vi "UDT_admittanceLibrary_PID.vi"() -> (3 "Unit Test Framework Results":T1)   [LabVIEW 2017]
doc: "Use this template to create a user-defined test VI. Define your test requirements and wire the results to the <b>Result (Test)</b> control. Do not modify the <b>Unit Test Framework Results</b> indicator."
uses:
  <vilib>/utf/common/utf_test_result_troll.ctl
  <vilib>/utf/common/utf_test_result.ctl
  <vilib>/utf/common/utf_test_result_failure.ctl
  <vilib>/utf/common/utf_test_comparison_operators.ctl
  <vilib>/utf/common/utf_vi_tag.ctl
  <vilib>/Control Software Solutions Ltd/UTF Helper/SubVIs/UTF Boolean Equals.vi
  <vilib>/Control Software Solutions Ltd/UTF Helper/SubVIs/UTF Double Equals.vi
  <vilib>/Control Software Solutions Ltd/UTF Helper/Unit Test Helper.lvlib
  RT/Admittance Controller/admittanceControllerLibrary.lvlib
  <vilib>/utf/NI_UnitTestFramework.lvlib
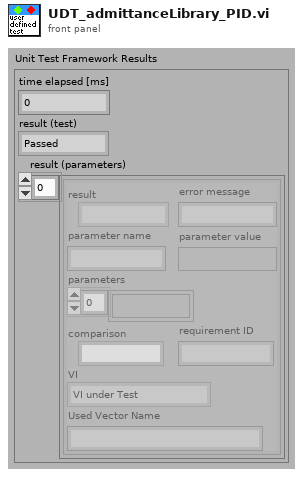
[diagram p1: front panel]
types:
  T1 = typedef "NI_UnitTestFramework.lvlib/utf_test_result_troll.ctl" = cluster{"time elapsed [ms]":u32, "result (test)":T2, "result (parameters)":T3[]}
  T2 = typedef "NI_UnitTestFramework.lvlib/utf_test_result.ctl" = enum16{"Passed", "Failed", "Error", "Skipped", "Not Processed"}
  T3 = typedef "NI_UnitTestFramework.lvlib/utf_test_result_failure.ctl" = cluster{"result":T2, "error message":string, "parameter name":string, "parameter value":variant, "parameters":variant[], "comparison":T4, "requirement ID":string, "VI":T5, "Used Vector Name":string}
  T4 = typedef "NI_UnitTestFramework.lvlib/utf_test_comparison_operators.ctl" = enum16{"=", "!=", ">", ">=", "<", "<=", "range", "symmetric tolerance", "asymmetric tolerance", "string contains", "string not contain", "array size", "string length", "array range", "by element", "array range (limit array)", "user-defined", "array contains", "array not contain", "vector length", "= (elm)", "!= (elm)", "= (case insensitive)", "!= (case insensitive)"}
  T5 = typedef "NI_UnitTestFramework.lvlib/utf_vi_tag.ctl" = enum16{"Setup VI", "VI under Test", "Teardown VI"}
  T6 = cluster{"proportional gain (Kc)":dbl, "integral time (Ti, min)":dbl, "derivative time (Td, min)":dbl}
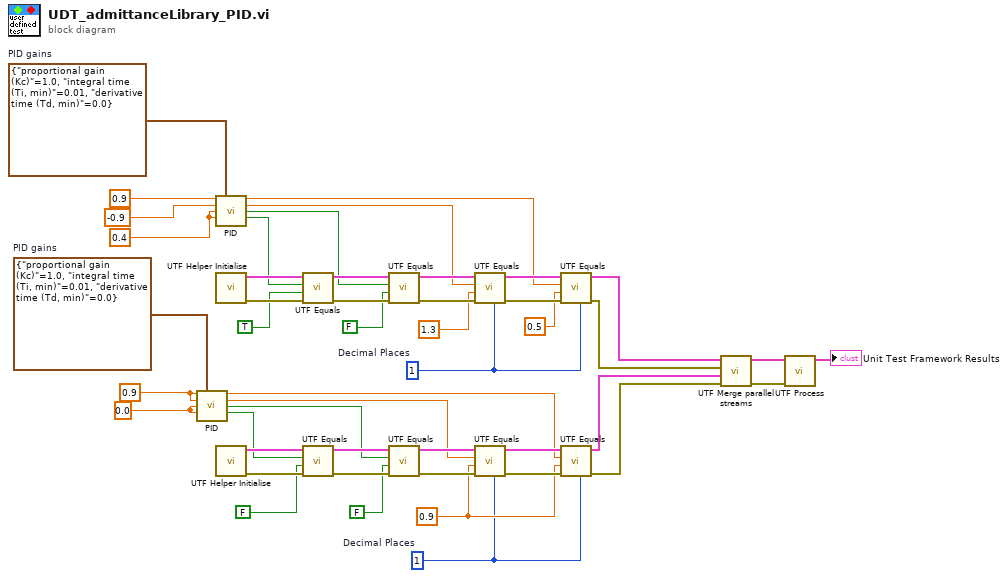
[diagram p0: block diagram]
diagram:
  w1 = u8 1  # Decimal Places
  w2 = u8 1  # Decimal Places
  w3 = 0.9
  w18 = 0.0
  w19 = 0.9
  w22 = 0.4
  w23 = T6 {"proportional gain (Kc)"=1.0, "integral time (Ti, min)"=0.01, "derivative time (Td, min)"=0.0}  # PID gains
  w24 = T6 {"proportional gain (Kc)"=1.0, "integral time (Ti, min)"=0.01, "derivative time (Td, min)"=0.0}  # PID gains
  n1 = call "PID.vi"("Des theta0"=w19, "PID gains"=w23, "Des theta1"=w19, "current theta0"=w18, "current theta1"=w18) -> ("U1"=w10:dbl, "U2"=w11:dbl, "Dir1"=w12:bool, "Dir2"=w13:bool)  [unwired: 6 in, 1 out]
  n2 = call "PID.vi"("Des theta0"=0.9, "PID gains"=w24, "Des theta1"=-0.9, "current theta0"=w22, "current theta1"=w22) -> ("U1"=w14:dbl, "U2"=w15:dbl, "Dir1"=w16:bool, "Dir2"=w17:bool)  [unwired: 6 in, 1 out]
  n3 = call <vilib>:"UTF Helper Initialise.vi"() -> ("error out"=w34:errorcluster, "results array"=w33:T3[])  [unwired: 10 in]
  n4 = call <vilib>:"UTF Helper Initialise.vi"() -> ("error out"=w25:errorcluster, "results array"=w32:T3[])  [unwired: 10 in]
  n5 = call-poly <vilib>:"UTF Equals.vi"("error in (no error)"=w34, "Test Value"=TRUE, "Input"=w17, "Input Results"=w33) -> ("error out"=w35:errorcluster, "Output Results"=w36:T3[])  [unwired: 6 in]
  n6 = call-poly <vilib>:"UTF Equals.vi"("error in (no error)"=w25, "Test Value"=FALSE, "Input"=w13, "Input Results"=w32) -> ("error out"=w26:errorcluster, "Output Results"=w31:T3[])  [unwired: 6 in]
  n7 = call-poly <vilib>:"UTF Equals.vi"("error in (no error)"=w35, "Test Value"=FALSE, "Input"=w16, "Input Results"=w36) -> ("error out"=w37:errorcluster, "Output Results"=w38:T3[])  [unwired: 6 in]
  n8 = call-poly <vilib>:"UTF Equals.vi"("error in (no error)"=w26, "Test Value"=FALSE, "Input"=w12, "Input Results"=w31) -> ("error out"=w27:errorcluster, "Output Results"=w30:T3[])  [unwired: 6 in]
  n9 = call-poly <vilib>:"UTF Equals.vi"("Decimal Places"=w2, "error in (no error)"=w37, "Test Value"=1.3, "Input"=w15, "Input Results"=w38) -> ("error out"=w40:errorcluster, "Output Results"=w39:T3[])  [unwired: 5 in]
  n10 = call-poly <vilib>:"UTF Equals.vi"("Decimal Places"=w1, "error in (no error)"=w27, "Test Value"=w3, "Input"=w11, "Input Results"=w30) -> ("error out"=w28:errorcluster, "Output Results"=w29:T3[])  [unwired: 5 in]
  n11 = call-poly <vilib>:"UTF Equals.vi"("Decimal Places"=w2, "error in (no error)"=w40, "Test Value"=0.5, "Input"=w14, "Input Results"=w39) -> ("error out"=w44:errorcluster, "Output Results"=w43:T3[])  [unwired: 5 in]
  n12 = call-poly <vilib>:"UTF Equals.vi"("Decimal Places"=w1, "error in (no error)"=w28, "Test Value"=w3, "Input"=w10, "Input Results"=w29) -> ("error out"=w41:errorcluster, "Output Results"=w42:T3[])  [unwired: 5 in]
  n13 = call <vilib>:"UTF Merge parallel streams.vi"("error in 2"=w41, "Results input 2"=w42, "error in 1"=w44, "Results input 1"=w43) -> ("error out"=w45:errorcluster, "Concatenated Results"=w46:T3[])  [unwired: 6 in]
  n14 = call <vilib>:"UTF Process.vi"("error in (no error)"=w45, "results array"=w46) -> ("Unit Test Framework Results"=→"Unit Test Framework Results":T1)  [unwired: 9 in]
